vi "ESP32LabViewComm.vi"() -> ()   [LabVIEW 2025]
uses:
  <vilib>/Instr/_visa.llb/VISA Configure Serial Port (Instr).vi
  <vilib>/addons/control/pid/pid.llb/PID (DBL).vi
  <vilib>/addons/control/pid/NI_PID_pid.lvlib
panel:
  out "Posicion Actual":dbl
  out "output":dbl format="%.2f"
  in  "PID gains":T1={"proportional gain (Kc)"=1.0, "integral time (Ti, min)"=0.01, "derivative time (Td, min)"=0.0} {"derivative time (Td, min)" format="%.3f"; "integral time (Ti, min)" format="%.3f"; "proportional gain (Kc)" format="%.3f"}
  in  "Set Point Grados":dbl
  out "PulsosIn":i32
  out "StringOut":string
  out "String In":string
  in  "stop":bool
  out "BOTON 3":bool
  out "BOTON 2":bool
  out "BOTON 1":bool
  in  "LED 3":bool
  in  "LED 2":bool
  in  "LED 1":bool
  in  "AZUL":i64(knob) scale=0.0..255.0
  out "POT 3":dbl(knob) scale=0.0..1023.0
  out "POT 2":dbl(knob) scale=0.0..1023.0
  out "POT1":dbl(knob) scale=0.0..1023.0
  in  "VISA resource name":refnum<visa-resource-name>
  # "I/O DIGITALES"
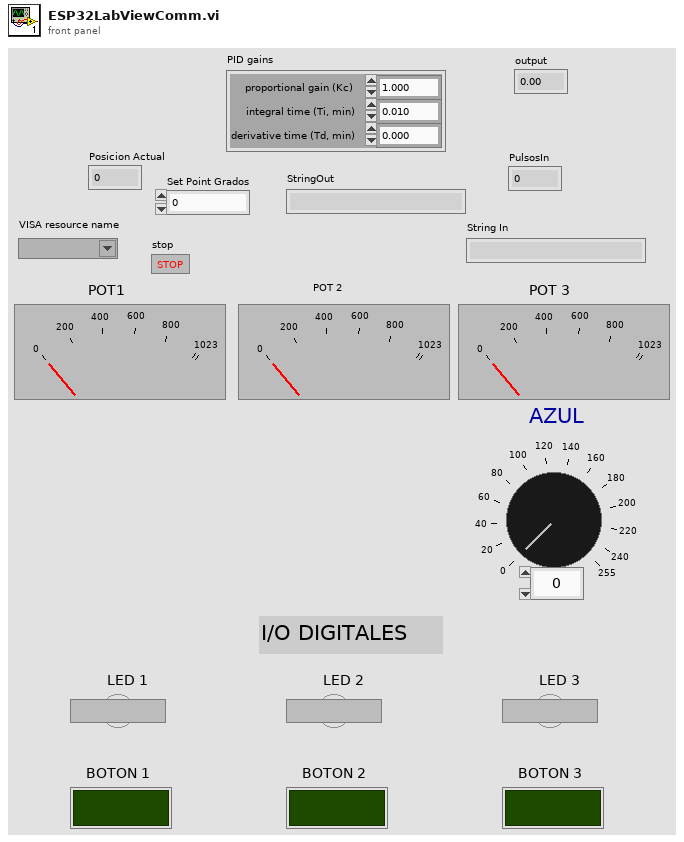
[diagram p1: front panel]
types:
  T1 = cluster{"proportional gain (Kc)":dbl, "integral time (Ti, min)":dbl, "derivative time (Td, min)":dbl}
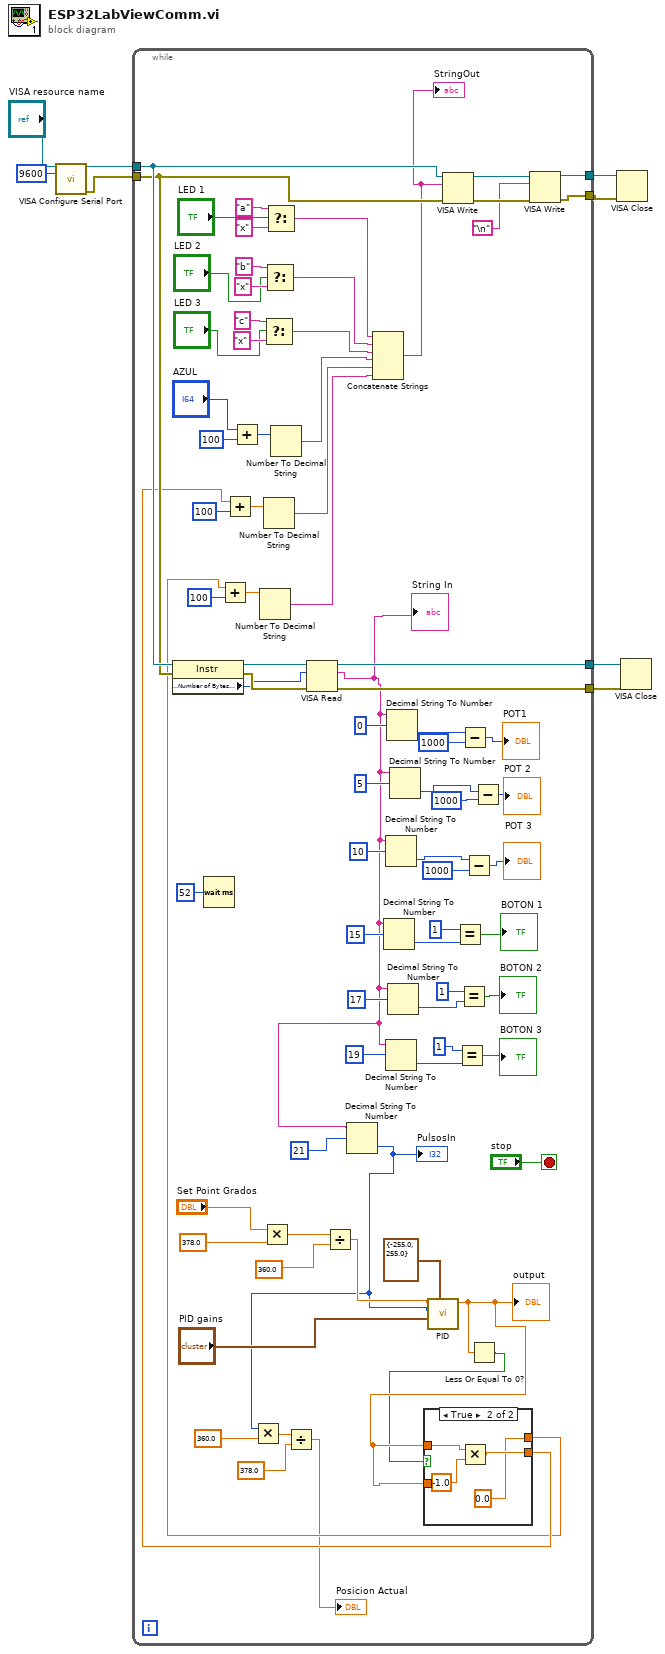
[diagram p0: block diagram]
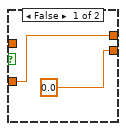
[diagram p2: hidden frame]
diagram:
  n1 = call-poly "VISA Configure Serial Port"("VISA resource name"="VISA resource name", "baud rate (9600)"=u32 9600) -> ("VISA resource name out"=w8:refnum<visa-resource-name>, "error out"=w7:errorcluster)  [unwired: 12 in]
  n2 = while {
    tunnel: w8 -> [w41]
    tunnel: w7 -> [w40]
    tunnel: [w29] -> w4
    tunnel: [w47] -> w3
    tunnel: [w46] -> w2
    tunnel: [w45] -> w1
    stop <- "stop" stop-if-true
    n3 = property class="Instr"(reference=w41, error in=w40) -> (reference out=w87:refnum<visa-resource-name>, error out=w86:errorcluster, "Serial Settings:Number of Bytes at Serial Port"=w85:u32)
    n4 = Wait (ms)(milliseconds to wait=u32 52) -> ()  [unwired: 1 out]
    n5 = Add(x="AZUL", y=i64 100) -> (x+y=w80:i64)
    n6 = Multiply(x="Set Point Grados", y=378.0) -> (x*y=w24:dbl)
    n7 = Select(t="c", s="LED 3", f="x") -> (s? t:f=w51:string)
    n8 = Select(t="b", s="LED 2", f="x") -> (s? t:f=w52:string)
    n9 = Select(t="a", s="LED 1", f="x") -> (s? t:f=w61:string)
    n10 = Number To Decimal String(number=w80) -> (decimal integer string=w50:string)  [unwired: 1 in]
    n11 = VISA Read(VISA resource name=w87, byte count=w85, error in (no error)=w86) -> (VISA resource name out=w46:refnum<visa-resource-name>, read buffer=w28:string, error out=w45:errorcluster)  [unwired: 1 out]
    "String In" <- w28
    n12 = Divide(x=w24, y=360.0) -> (x/y=w20:dbl)
    n13 = Decimal String To Number(string=w28, offset=21) -> (number=w12:i32)  [unwired: 1 in, 1 out]
    "PulsosIn" <- w12
    n14 = Multiply(x=w12, y=360.0) -> (x*y=w11:dbl)
    n15 = Divide(x=w11, y=378.0) -> (x/y=→"Posicion Actual":dbl)
    n16 = Decimal String To Number(string=w28, offset=15 ("offset (0)")) -> (number=w37:i32)  [unwired: 1 in, 1 out]
    n17 = Decimal String To Number(string=w28, offset=10) -> (number=w65:i32)  [unwired: 1 in, 1 out]
    n18 = Decimal String To Number(string=w28, offset=19 ("offset (0)")) -> (number=w31:i32)  [unwired: 1 in, 1 out]
    n19 = Decimal String To Number(string=w28, offset=0) -> (number=w72:i32)  [unwired: 1 in, 1 out]
    n20 = Decimal String To Number(string=w28, offset=17 ("offset (0)")) -> (number=w33:i32)  [unwired: 1 in, 1 out]
    n21 = Decimal String To Number(string=w28, offset=5) -> (number=w68:i32)  [unwired: 1 in, 1 out]
    n22 = call-poly <vilib>:"PID.vi"("output range"=cluster{"output high":dbl, "output low":dbl} {"output high"=-255.0, "output low"=255.0}, "PID gains"="PID gains", "process variable"=w12, "setpoint"=w20) -> ("output"=w15:dbl)  [unwired: 6 in, 1 out]
    "output" <- w15
    n23 = Equal?(x=1 ("y"), y=w37) -> (x = y?=→"BOTON 1":bool)
    n24 = Equal?(x=1 ("y"), y=w31) -> (x = y?=→"BOTON 3":bool)
    n25 = Equal?(x=1 ("y"), y=w33) -> (x = y?=→"BOTON 2":bool)
    n26 = Subtract(x=w72, y=1000) -> (x-y=→"POT1":i32)
    n27 = Subtract(x=w65, y=1000) -> (x-y=→"POT 3":i32)
    n28 = Less Or Equal To 0?(x=w15) -> (x <= 0?=w14:bool)
    n29 = case shown="True" w14 {
      tunnel: w15 -> [_ w92]
      tunnel: [0.0 w91] -> w17
      tunnel: [w88 0.0] -> w16
      tunnel: w15 -> [w88 _]
      frame False {
      }
      frame True {
        n30 = Multiply(x=w92, y=-1.0) -> (x*y=w91:dbl)
      }
    }
    n31 = Add(x=w16, y=i64 100) -> (x+y=w75:dbl)
    n32 = Add(x=w17, y=i64 100) -> (x+y=w76:dbl)
    n33 = Number To Decimal String(number=w75) -> (decimal integer string=w48:string)  [unwired: 1 in]
    n34 = Number To Decimal String(number=w76) -> (decimal integer string=w49:string)  [unwired: 1 in]
    n35 = Concatenate Strings(w61, w52, w51, w50, w49, w48) -> (w18:string)
    "StringOut" <- w18
    n36 = VISA Write(VISA resource name=w41, write buffer=w18, error in (no error)=w40) -> (VISA resource name out=w19:refnum<visa-resource-name>, error out=w64:errorcluster)  [unwired: 1 out]
    n37 = Subtract(x=w68, y=1000) -> (x-y=→"POT 2":i32)
    n38 = VISA Write(VISA resource name=w19, write buffer="\n", error in (no error)=w64) -> (VISA resource name out=w29:refnum<visa-resource-name>, error out=w47:errorcluster)  [unwired: 1 out]
  }
  n39 = VISA Close(VISA resource name=w4, error in (no error)=w3) -> ()  [unwired: 1 out]
  n40 = VISA Close(VISA resource name=w2, error in (no error)=w1) -> ()  [unwired: 1 out]
